vi "SaveSystemConfigurationUI.vi"(8 "error in (no error)":errorcluster, 11 "HardwareSetup_modle001:HardwareSetup_modle001":refnum<class "HardwareSetup_model001.lvclass">) -> (0 "error out":errorcluster, 3 "HardwareSetup_modle001:HardwareSetup_modle001":refnum<class "HardwareSetup_model001.lvclass">)   [LabVIEW 2019, in "HardwareSetup_model001.lvlib" / "HardwareSetup_model001.lvclass"]
uses:
  HardwareSetup_model001.lvclass
  C:/Program Files (x86)/National Instruments/LabVIEW 2019/vi.lib/NI/Event Source Actor/Event Source/Event Source/Event Source.lvclass
  HardwareSetup_model001.lvclass/HardwareSetup_model001.ctl
  SystemSetup/SystemSetup/SystemConfiguration.lvclass
  C:/Program Files (x86)/National Instruments/LabVIEW 2019/vi.lib/NI/Event Source Actor/Event Source/Event/Event.lvclass
  <vilib>/NI/Event Source Actor/Event Source/Event/Event.lvclass/Event.ctl
  SystemSetup/SystemSetup/SystemSetup.lvclass
  <vilib>/NI/Event Source Actor/Event Source/Event/Event.lvclass
  <vilib>/NI/Event Source Actor/Event Source/Event Source/Event Source.lvclass
  <vilib>/Utility/config.llb/NI_LVConfig.lvlib
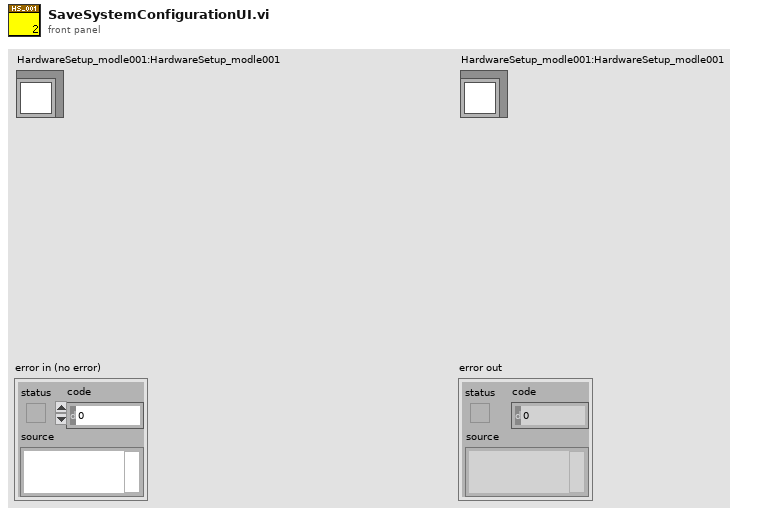
[diagram p1: front panel]
types:
  T1 = typedef "HardwareSetup_model001.lvlib/LIN.ctl" = cluster{"LIN 1":cluster{"Instrument model":string, "Port":string, "Baud rate":i32, "ID":i32, "Terminal":bool}, "LIN 2":cluster{"Instrument model":string, "Port":string, "Baud rate":i32, "ID":i32, "Terminal":bool}, "LIN 3":cluster{"Instrument model":string, "Port":string, "Baud rate":i32, "ID":i32, "Terminal":bool}, "LIN 4":cluster{"Instrument model":string, "Port":string, "Baud rate":i32, "ID":i32, "Terminal":bool}}
  T2 = typedef "HardwareSetup_model001.lvlib/Digital IO.ctl" = cluster{"Digital IO 1":cluster{"SerialPort":string, "Baud rate":i32, "Address":string, "ID":i32, "Port":i32, "Instrument model":string}, "Digital IO 2":cluster{"SerialPort":string, "Baud rate":i32, "Address":string, "ID":i32, "Port":i32, "Instrument model":string}, "Digital IO 3":cluster{"SerialPort":string, "Baud rate":i32, "Address":string, "ID":i32, "Port":i32, "Instrument model":string}, "Digital IO 4":cluster{"SerialPort":string, "Baud rate":i32, "Address":string, "ID":i32, "Port":i32, "Instrument model":string}}
  T3 = typedef "HardwareSetup_model001.lvlib/DMM.ctl" = cluster{"DMM 1":cluster{"SerialPort":string, "Baud rate":i32, "Address":string, "ID":i32, "Port":i32, "Instrument model":string}, "DMM 2":cluster{"SerialPort":string, "Baud rate":i32, "Address":string, "ID":i32, "Port":i32, "Instrument model":string}, "DMM 3":cluster{"SerialPort":string, "Baud rate":i32, "Address":string, "ID":i32, "Port":i32, "Instrument model":string}, "DMM 4":cluster{"SerialPort":string, "Baud rate":i32, "Address":string, "ID":i32, "Port":i32, "Instrument model":string}}
  T4 = typedef "HardwareSetup_model001.lvlib/Oscilloscope.ctl" = cluster{"Oscilloscope 1":cluster{"SerialPort":string, "Baud rate":i32, "Address":string, "ID":i32, "Port":i32, "Instrument model":string}, "Oscilloscope 2":cluster{"SerialPort":string, "Baud rate":i32, "Address":string, "ID":i32, "Port":i32, "Instrument model":string}, "Oscilloscope 3":cluster{"SerialPort":string, "Baud rate":i32, "Address":string, "ID":i32, "Port":i32, "Instrument model":string}, "Oscilloscope 4":cluster{"SerialPort":string, "Baud rate":i32, "Address":string, "ID":i32, "Port":i32, "Instrument model":string}}
  T5 = typedef "HardwareSetup_model001.lvlib/PLC.ctl" = cluster{"PLC 1":cluster{"SerialPort":string, "Baud rate":i32, "Address":string, "ID":i32, "Port":i32, "Instrument model":string}}
  T6 = typedef "HardwareSetup_model001.lvlib/ElectronicLoad.ctl" = cluster{"ElectronicLoad 1":cluster{"SerialPort":string, "Baud rate":i32, "Address":string, "ID":i32, "Port":i32, "Instrument model":string}, "ElectronicLoad 2":cluster{"SerialPort":string, "Baud rate":i32, "Address":string, "ID":i32, "Port":i32, "Instrument model":string}, "ElectronicLoad 3":cluster{"SerialPort":string, "Baud rate":i32, "Address":string, "ID":i32, "Port":i32, "Instrument model":string}, "ElectronicLoad 4":cluster{"SerialPort":string, "Baud rate":i32, "Address":string, "ID":i32, "Port":i32, "Instrument model":string}}
  T7 = typedef "HardwareSetup_model001.lvlib/PowerSupply.ctl" = cluster{"PowerSupply 1":cluster{"SerialPort":string, "Baud rate":i32, "Address":string, "ID":i32, "Port":i32, "Instrument model":string}, "PowerSupply 2":cluster{"SerialPort":string, "Baud rate":i32, "Address":string, "ID":i32, "Port":i32, "Instrument model":string}, "PowerSupply 3":cluster{"SerialPort":string, "Baud rate":i32, "Address":string, "ID":i32, "Port":i32, "Instrument model":string}, "PowerSupply 4":cluster{"SerialPort":string, "Baud rate":i32, "Address":string, "ID":i32, "Port":i32, "Instrument model":string}}
  T8 = typedef "HardwareSetup_model001.lvlib/CAN.ctl" = cluster{"CAN 1":cluster{"Instrument model":string, "Port":string, "Baud rate":i32, "ID":i32, "Terminal":bool}, "CAN 2":cluster{"Instrument model":string, "Port":string, "Baud rate":i32, "ID":i32, "Terminal":bool}, "CAN 3":cluster{"Instrument model":string, "Port":string, "Baud rate":i32, "ID":i32, "Terminal":bool}, "CAN 4":cluster{"Instrument model":string, "Port":string, "Baud rate":i32, "ID":i32, "Terminal":bool}}
  T9 = typedef "HardwareSetup_model001.lvlib/Programming.ctl" = cluster{"Programming 1":cluster{"Test Image":string, "Address":string, "Port":i32, "Instrument model":string, "Final Image":string}, "Programming 2":cluster{"Test Image":string, "Address":string, "Port":i32, "Instrument model":string, "Final Image":string}}
  T10 = typedef "HardwareSetup_model001.lvlib/Scanner.ctl" = cluster{"Scanner 1":cluster{"SerialPort":string, "Baud rate":i32, "Address":string, "ID":i32, "Port":i32, "Instrument model":string}, "Scanner 2":cluster{"SerialPort":string, "Baud rate":i32, "Address":string, "ID":i32, "Port":i32, "Instrument model":string}, "Scanner 3":cluster{"SerialPort":string, "Baud rate":i32, "Address":string, "ID":i32, "Port":i32, "Instrument model":string}, "Scanner 4":cluster{"SerialPort":string, "Baud rate":i32, "Address":string, "ID":i32, "Port":i32, "Instrument model":string}}
  T11 = cluster{"LIN":T1, "Digital IO":T2, "DMM":T3, "Oscilloscope":T4, "PLC":T5, "ElectronicLoad":T6, "PowerSupply":T7, "CAN":T8, "Programming":T9, "Scanner":T10}
  T12 = typedef "HardwareSetup_bench001.lvlib/ElectronicLoad.ctl" = cluster{"ElectronicLoad 1":cluster{"SerialPort":string, "Baud rate":i32, "Address":string, "ID":i32, "Port":i32, "Instrument model":string}, "ElectronicLoad 2":cluster{"SerialPort":string, "Baud rate":i32, "Address":string, "ID":i32, "Port":i32, "Instrument model":string}, "ElectronicLoad 3":cluster{"SerialPort":string, "Baud rate":i32, "Address":string, "ID":i32, "Port":i32, "Instrument model":string}, "ElectronicLoad 4":cluster{"SerialPort":string, "Baud rate":i32, "Address":string, "ID":i32, "Port":i32, "Instrument model":string}}
  T13 = typedef "HardwareSetup_bench001.lvlib/PowerSupply.ctl" = cluster{"PowerSupply 1":cluster{"SerialPort":string, "Baud rate":i32, "Address":string, "ID":i32, "Port":i32, "Instrument model":string}, "PowerSupply 2":cluster{"SerialPort":string, "Baud rate":i32, "Address":string, "ID":i32, "Port":i32, "Instrument model":string}, "PowerSupply 3":cluster{"SerialPort":string, "Baud rate":i32, "Address":string, "ID":i32, "Port":i32, "Instrument model":string}, "PowerSupply 4":cluster{"SerialPort":string, "Baud rate":i32, "Address":string, "ID":i32, "Port":i32, "Instrument model":string}}
  T14 = typedef "HardwareSetup_modle001.lvlib/CAN.ctl" = cluster{"CAN 1":cluster{"Instrument model":string, "SerialPort":string, "Baud rate":i32, "ID":i32, "Terminal":bool}, "CAN 2":cluster{"Instrument model":string, "SerialPort":string, "Baud rate":i32, "ID":i32, "Terminal":bool}, "CAN 3":cluster{"Instrument model":string, "SerialPort":string, "Baud rate":i32, "ID":i32, "Terminal":bool}, "CAN 4":cluster{"Instrument model":string, "SerialPort":string, "Baud rate":i32, "ID":i32, "Terminal":bool}}
  T15 = typedef "HardwareSetup_bench001.lvlib/Programming.ctl" = cluster{"DMM 1":cluster{"Test Image":string, "Address":string, "Port":i32, "Instrument model":string, "Final Image":string}, "DMM 2":cluster{"Test Image":string, "Address":string, "Port":i32, "Instrument model":string, "Final Image":string}}
  T16 = typedef "HardwareSetup_bench001.lvlib/Scanner.ctl" = cluster{"Scanner 1":cluster{"SerialPort":string, "Baud rate":i32, "Address":string, "ID":i32, "Port":i32, "Instrument model":string}, "Scanner 2":cluster{"SerialPort":string, "Baud rate":i32, "Address":string, "ID":i32, "Port":i32, "Instrument model":string}, "Scanner 3":cluster{"SerialPort":string, "Baud rate":i32, "Address":string, "ID":i32, "Port":i32, "Instrument model":string}, "Scanner 4":cluster{"SerialPort":string, "Baud rate":i32, "Address":string, "ID":i32, "Port":i32, "Instrument model":string}}
  T17 = typedef "HardwareSetup_modle001.lvlib/LIN.ctl" = cluster{"LIN 1":cluster{"Instrument model":string, "SerialPort":string, "Baud rate":i32, "ID":i32, "Terminal":bool}, "LIN 2":cluster{"Instrument model":string, "SerialPort":string, "Baud rate":i32, "ID":i32, "Terminal":bool}, "LIN 3":cluster{"Instrument model":string, "SerialPort":string, "Baud rate":i32, "ID":i32, "Terminal":bool}, "LIN 4":cluster{"Instrument model":string, "SerialPort":string, "Baud rate":i32, "ID":i32, "Terminal":bool}}
  T18 = typedef "HardwareSetup_bench001.lvlib/Digital IO.ctl" = cluster{"Digital IO 1":cluster{"SerialPort":string, "Baud rate":i32, "Address":string, "ID":i32, "Port":i32, "Instrument model":string}, "Digital IO 2":cluster{"SerialPort":string, "Baud rate":i32, "Address":string, "ID":i32, "Port":i32, "Instrument model":string}, "Digital IO 3":cluster{"SerialPort":string, "Baud rate":i32, "Address":string, "ID":i32, "Port":i32, "Instrument model":string}, "Digital IO 4":cluster{"SerialPort":string, "Baud rate":i32, "Address":string, "ID":i32, "Port":i32, "Instrument model":string}}
  T19 = typedef "HardwareSetup_bench001.lvlib/DMM.ctl" = cluster{"DMM 1":cluster{"SerialPort":string, "Baud rate":i32, "Address":string, "ID":i32, "Port":i32, "Instrument model":string}, "DMM 2":cluster{"SerialPort":string, "Baud rate":i32, "Address":string, "ID":i32, "Port":i32, "Instrument model":string}, "DMM 3":cluster{"SerialPort":string, "Baud rate":i32, "Address":string, "ID":i32, "Port":i32, "Instrument model":string}, "DMM 4":cluster{"SerialPort":string, "Baud rate":i32, "Address":string, "ID":i32, "Port":i32, "Instrument model":string}}
  T20 = typedef "HardwareSetup_bench001.lvlib/Oscilloscope.ctl" = cluster{"Oscilloscope 1":cluster{"SerialPort":string, "Baud rate":i32, "Address":string, "ID":i32, "Port":i32, "Instrument model":string}, "Oscilloscope 2":cluster{"SerialPort":string, "Baud rate":i32, "Address":string, "ID":i32, "Port":i32, "Instrument model":string}, "Oscilloscope 3":cluster{"SerialPort":string, "Baud rate":i32, "Address":string, "ID":i32, "Port":i32, "Instrument model":string}, "Oscilloscope 4":cluster{"SerialPort":string, "Baud rate":i32, "Address":string, "ID":i32, "Port":i32, "Instrument model":string}}
  T21 = typedef "HardwareSetup_bench001.lvlib/PLC.ctl" = cluster{"PLC 1":cluster{"SerialPort":string, "Baud rate":i32, "Address":string, "ID":i32, "Port":i32, "Instrument model":string}}
  T22 = typedef "NI_LVConfig.lvlib/Config Data RefNum.ctl" = refnum<k1>
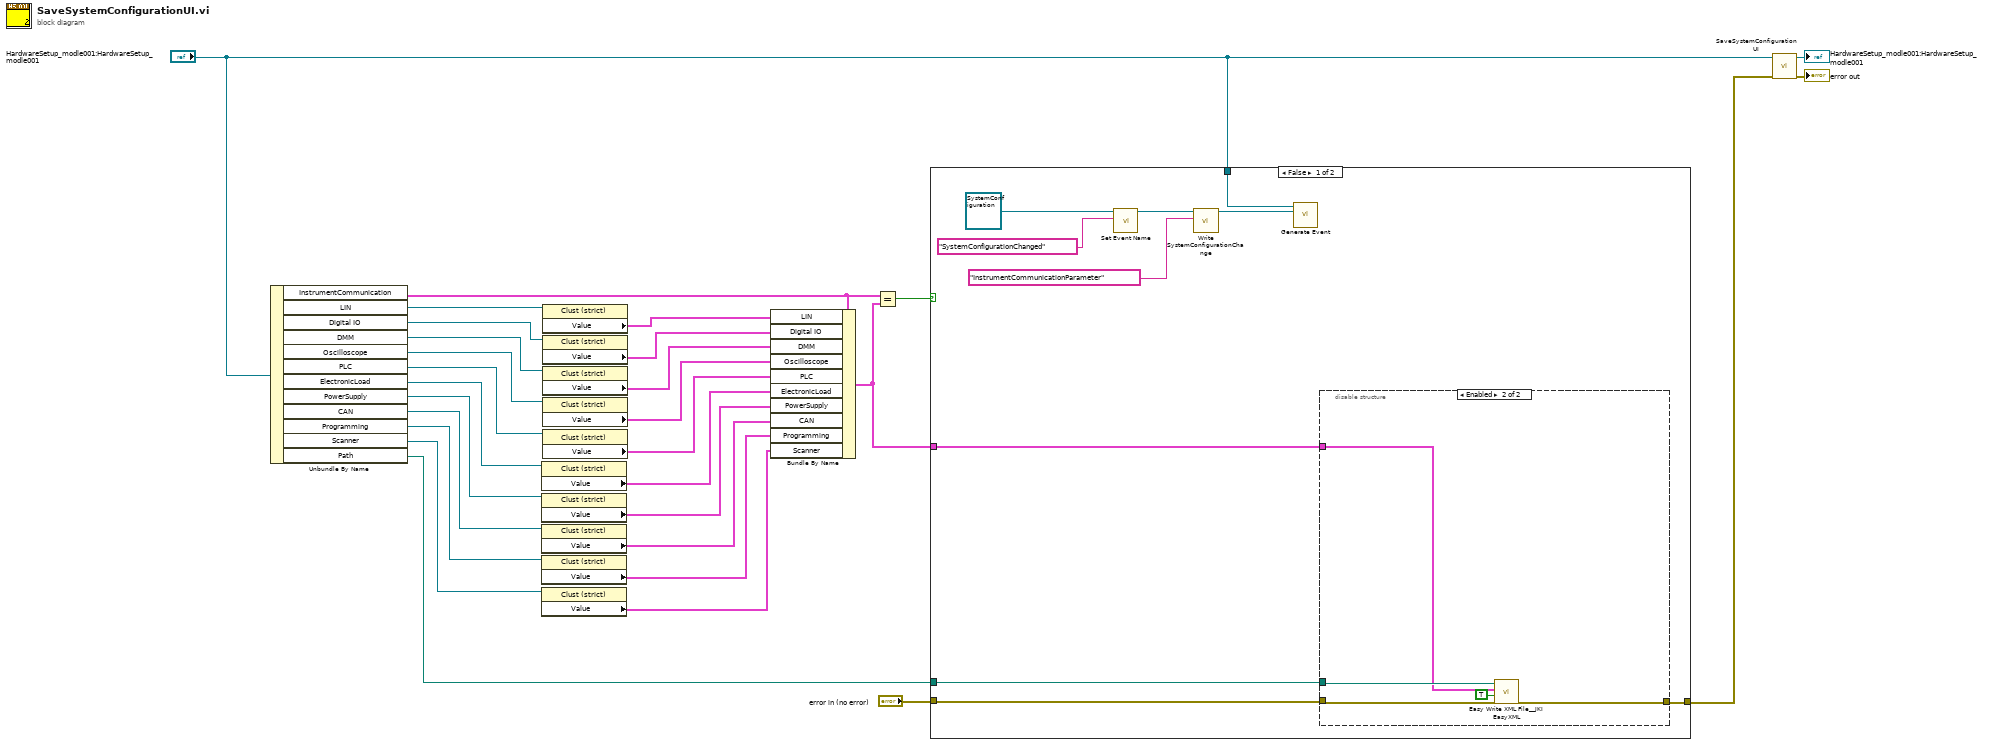
[diagram p0: block diagram]
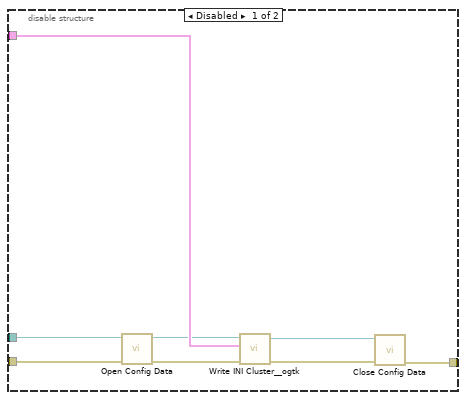
[diagram p2: hidden frame]
diagram:
  n1 = Unbundle By Name("HardwareSetup_modle001:HardwareSetup_modle001") -> ("InstrumentCommunication"=w15:T11, "LIN"=w27:refnum<vi>, "Digital IO"=w25:refnum<vi>, "DMM"=w24:refnum<vi>, "Oscilloscope"=w23:refnum<vi>, "PLC"=w22:refnum<vi>, "ElectronicLoad"=w13:refnum<vi>, "PowerSupply"=w12:refnum<vi>, "CAN"=w11:refnum<vi>, "Programming"=w10:refnum<vi>, "Scanner"=w9:refnum<vi>, "Path"=w8:path)
  n2 = property class="Clust (strict)"(reference=w13) -> ("Value"=w7:T12)  [unwired: 1 in, 2 out]
  n3 = property class="Clust (strict)"(reference=w12) -> ("Value"=w6:T13)  [unwired: 1 in, 2 out]
  n4 = property class="Clust (strict)"(reference=w11) -> ("Value"=w5:T14)  [unwired: 1 in, 2 out]
  n5 = property class="Clust (strict)"(reference=w10) -> ("Value"=w4:T15)  [unwired: 1 in, 2 out]
  n6 = property class="Clust (strict)"(reference=w9) -> ("Value"=w3:T16)  [unwired: 1 in, 2 out]
  n7 = property class="Clust (strict)"(reference=w27) -> ("Value"=w21:T17)  [unwired: 1 in, 2 out]
  n8 = property class="Clust (strict)"(reference=w25) -> ("Value"=w20:T18)  [unwired: 1 in, 2 out]
  n9 = property class="Clust (strict)"(reference=w24) -> ("Value"=w19:T19)  [unwired: 1 in, 2 out]
  n10 = property class="Clust (strict)"(reference=w23) -> ("Value"=w18:T20)  [unwired: 1 in, 2 out]
  n11 = property class="Clust (strict)"(reference=w22) -> ("Value"=w17:T21)  [unwired: 1 in, 2 out]
  n12 = Bundle By Name(cluster=w15, "LIN"=w21, "Digital IO"=w20, "DMM"=w19, "Oscilloscope"=w18, "PLC"=w17, "ElectronicLoad"=w7, "PowerSupply"=w6, "CAN"=w5, "Programming"=w4, "Scanner"=w3) -> (w16:T11)
  n13 = Equal?(x=w15, y=w16) -> (x = y?=w26:bool)
  n14 = case shown="False" w26 {
    tunnel: "error in (no error)" -> [w39 w53]
    tunnel: [w38 w53] -> w1
    tunnel: w8 -> [w37 _]
    tunnel: w16 -> [w36 _]
    tunnel: "HardwareSetup_modle001:HardwareSetup_modle001" -> [w31 _]
    frame False {
      n15 = call <vilib>:"Set Event Name.vi"("Name (Generic)"="SystemConfigurationChanged", "Event In"=refnum<class "SystemConfiguration.lvclass"> refnum ("SystemSetup.lvlib:SystemConfiguration.lvclass")) -> ("Event Out"=w33:refnum<class "SystemConfiguration.lvclass">)  [unwired: 9 in]
      n16 = call-dynamic "Write SystemConfigurationChange.vi"("SystemConfigurationChange"="InstrumentCommunicationParameter", "SystemConfiguration in"=w33) -> ("SystemConfiguration out"=w32:refnum<class "SystemConfiguration.lvclass">)  [unwired: 8 in, 1 out]
      n17 = call <vilib>:"Generate Event.vi"("Event"=w32, "Event Source In"=w31) -> ()  [unwired: 8 in, 2 out]
      n18 = disable-structure shown="Enabled" {
        disable-tunnel: w39 -> [w47 w51]
        disable-tunnel: [w46 w49] -> w38
        disable-tunnel: w37 -> [w45 w52]
        disable-tunnel: w36 -> [w44 w50]
        frame Disabled {
          n19 = call <vilib>:"Open Config Data.vi"("error in (no error)"=w47, "configuration file path"=w45) -> ("error out"=w42:errorcluster, "refnum"=w43:T22)  [unwired: 7 in, 1 out]
          n20 = call <userlib>:"Write INI Cluster__ogtk.vi"("error in (no error)"=w42, "INI Fomatted Cluster"=w44, "refnum"=w43) -> ("error out"=w40:errorcluster, "dup refnum"=w41:T22)  [unwired: 7 in]
          n21 = call <vilib>:"Close Config Data.vi"("error in (no error)"=w40, "refnum"=w41) -> ("error out"=w46:errorcluster)  [unwired: 8 in, 1 out]
        }
        frame Enabled {
          n22 = call <vilib>:"Easy Write XML File__JKI EasyXML.vi"("error in (no error)"=w51, "Overwrite File? (false)"=TRUE, "LabVIEW Data"=w50, "XML File Path"=w52) -> ("error out"=w49:errorcluster)  [unwired: 6 in, 1 out]
        }
      }
    }
    frame True {
    }
  }
  n23 = call-parent "SaveSystemConfigurationUI.vi"("error in (no error)"=w1, "SystemSetup in"="HardwareSetup_modle001:HardwareSetup_modle001") -> ("error out"=→"error out":errorcluster, "SystemSetup out"=→"HardwareSetup_modle001:HardwareSetup_modle001":refnum<class "HardwareSetup_model001.lvclass">)  [unwired: 8 in]
